vi "find steer angle errors.vi"(10 "Desired Motion":T1, 11 "Actual Angles":T1) -> (3 "Commanded Motion":T1)   [LabVIEW 2018]
uses:
  Robot Pivot Motion Commands.ctl
  Pivot Motor Commands.ctl
  Robot Drive Mode.ctl
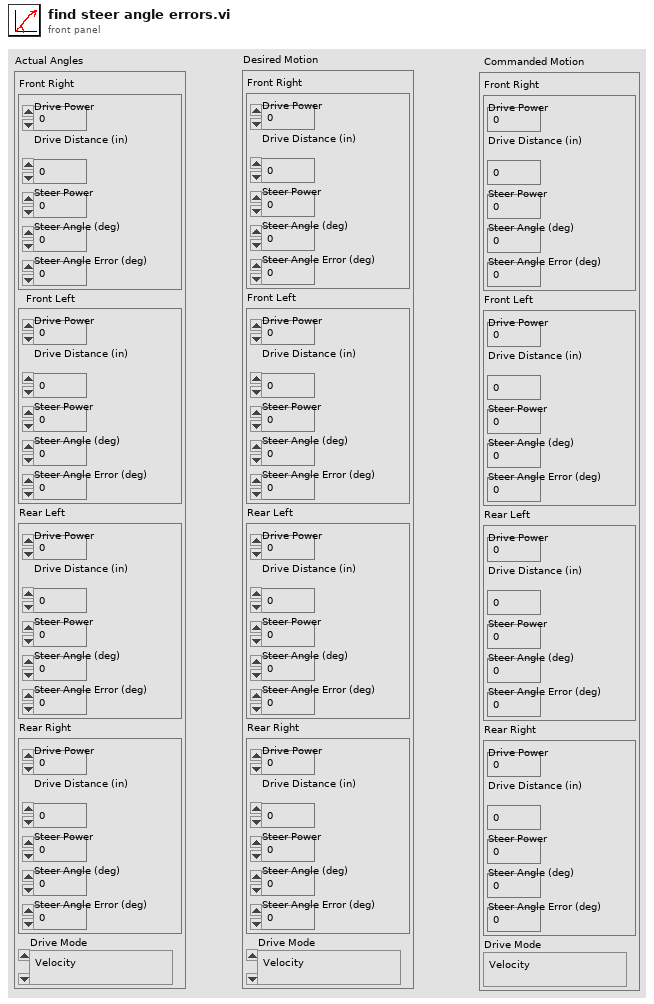
[diagram p1: front panel]
types:
  T1 = typedef "Robot Pivot Motion Commands.ctl" = cluster{"Front Right":T2, "Front Left":T2, "Rear Left":T2, "Rear Right":T2, "Drive Mode":T3}
  T2 = typedef "Pivot Motor Commands.ctl" = cluster{"Drive Power":dbl, "Drive Distance (in)":dbl, "Steer Power":dbl, "Steer Angle (deg)":dbl, "Steer Angle Error (deg)":dbl}
  T3 = typedef "Robot Drive Mode.ctl" = enum16{"Velocity", "Distance"}
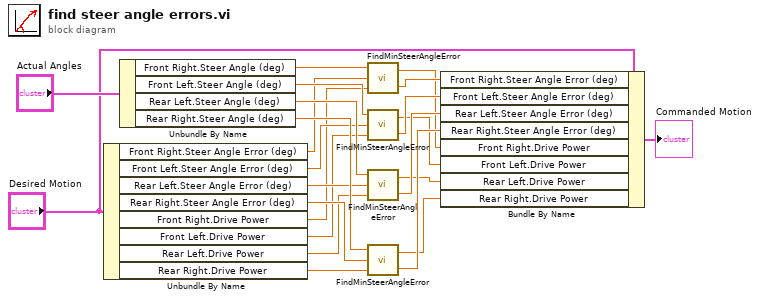
[diagram p0: block diagram]
diagram:
  n1 = Unbundle By Name("Desired Motion") -> ("Front Right.Steer Angle Error (deg)"=w18:dbl, "Front Left.Steer Angle Error (deg)"=w17:dbl, "Rear Left.Steer Angle Error (deg)"=w16:dbl, "Rear Right.Steer Angle Error (deg)"=w15:dbl, "Front Right.Drive Power"=w12:dbl, "Front Left.Drive Power"=w11:dbl, "Rear Left.Drive Power"=w10:dbl, "Rear Right.Drive Power"=w9:dbl)
  n2 = Unbundle By Name("Actual Angles") -> ("Front Right.Steer Angle (deg)"=w22:dbl, "Front Left.Steer Angle (deg)"=w21:dbl, "Rear Left.Steer Angle (deg)"=w20:dbl, "Rear Right.Steer Angle (deg)"=w19:dbl)
  n3 = call "FindMinSteerAngleError.vi"("Motor Power"=w12, "Desired Angle"=w18, "Actual Angle"=w22) -> ("Angle Error"=w8:dbl, "Motor Power"=w4:dbl)
  n4 = call "FindMinSteerAngleError.vi"("Motor Power"=w11, "Desired Angle"=w17, "Actual Angle"=w21) -> ("Angle Error"=w7:dbl, "Motor Power"=w3:dbl)
  n5 = call "FindMinSteerAngleError.vi"("Motor Power"=w10, "Desired Angle"=w16, "Actual Angle"=w20) -> ("Angle Error"=w6:dbl, "Motor Power"=w2:dbl)
  n6 = call "FindMinSteerAngleError.vi"("Motor Power"=w9, "Desired Angle"=w15, "Actual Angle"=w19) -> ("Angle Error"=w5:dbl, "Motor Power"=w1:dbl)
  n7 = Bundle By Name(cluster="Desired Motion", "Front Right.Steer Angle Error (deg)"=w8, "Front Left.Steer Angle Error (deg)"=w7, "Rear Left.Steer Angle Error (deg)"=w6, "Rear Right.Steer Angle Error (deg)"=w5, "Front Right.Drive Power"=w4, "Front Left.Drive Power"=w3, "Rear Left.Drive Power"=w2, "Rear Right.Drive Power"=w1) -> (→"Commanded Motion":T1)
